vi "Get JSON.vi"(11 "ConfigFromJSON in":refnum<class "Config Hardcoded.lvclass">) -> (2 "<JSON>":string, 3 "ConfigFromJSON out":refnum<class "Config Hardcoded.lvclass">)   [LabVIEW 2024, in "PCAN.lvlib" / "Config Hardcoded.lvclass"]
uses:
  Config Hardcoded.lvclass
  Config Hardcoded.lvclass/Config Hardcoded.ctl
panel:
  out "String":string
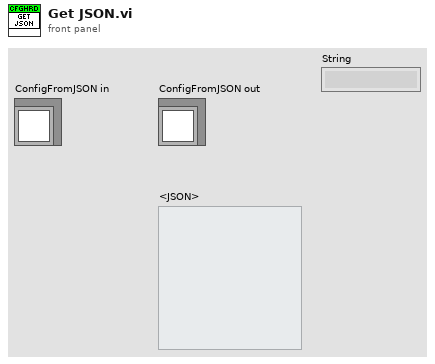
[diagram p1: front panel]
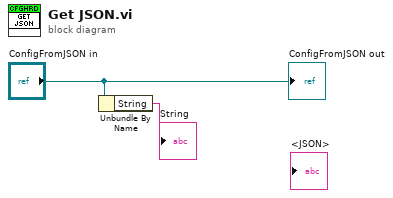
[diagram p0: block diagram]
diagram:
  n1 = Unbundle By Name("ConfigFromJSON in") -> ("String"=→"String":string)
  "ConfigFromJSON out" <- "ConfigFromJSON in"
